vi "reg_visu check 20 client.vi"() -> ()   [LabVIEW 2019]
uses:
  Heating/Global stop.vi
panel:
  out "Array 3":errorcluster[](array[cluster])
  in  "Array 2":string[](array[string])=["GM1", "GM2"]
  out "Errors":errorcluster[](array[cluster])
  out "Progress 3":i32(slide) scale=0.0..20.0
  in  "Stop":bool
  in  "Array":string[](array[string])=["GM1", "GM2", "GM3", "GM4", "GM5", "GM6", "GM7", "GM8", "GM9", "GM10", "GM11", "GM12", "GM13", "GM14", "GM15", "GM16", "GM17", "GM18", "GM19", "GM20"]
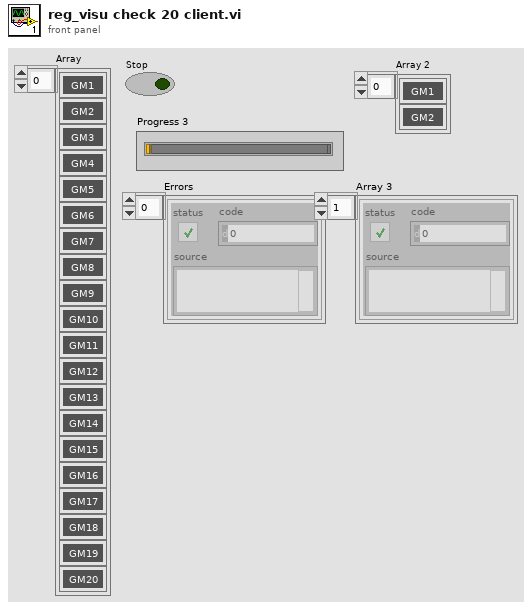
[diagram p1: front panel]
types:
  T1 = enum32{"Invalid", "Standard", "Closed", "Hidden", "Minimized", "Maximized"}
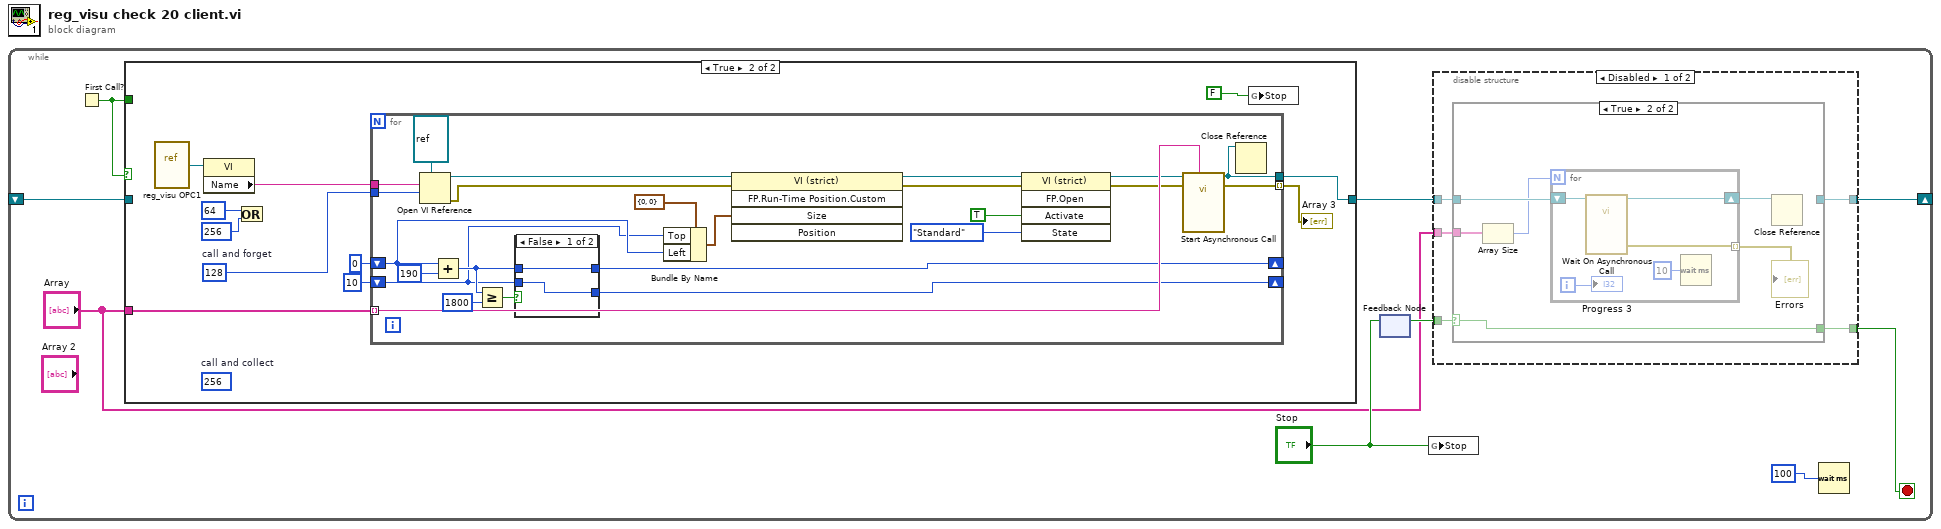
[diagram p0: block diagram]
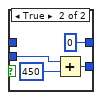
[diagram p5: hidden frame]
diagram:
  n1 = while {
    shift-right: [w5] -> _
    shift-left: _ -> [w7]
    stop <- w2 stop-if-true
    n2 = First Call?() -> (First Call?: T/F=w8:bool)
    n3 = case shown="True" w8 {
      tunnel: w8 -> [_ _]
      tunnel: "Array" -> [_ w39]
      tunnel: [w30 w41] -> w6
      tunnel: w7 -> [w30 _]
      frame False {
      }
      frame True {
        w32 = 128  # call and forget
        (unwired) 256  # call and collect
        n4 = vi-ref "reg_visu OPC1.vi"() -> (w40:refnum<vi>)
        n5 = property class="VI"(reference=w40) -> ("Name"=w33:string)  [unwired: 1 in, 2 out]
        n6 = Or(x=64 ("options"), y=256 ("options")) -> ()  [unwired: 1 out]
        n7 = for {
          tunnel: w39 -> [w65] mode=indexing
          shift-right: [w57] -> _
          shift-left: 0 ("x") -> [w50]
          shift-right: [w56] -> _
          shift-left: 10 ("x") -> [w49]
          tunnel: [w43] -> w41
          tunnel: w32 -> [w47]
          tunnel: w33 -> [w46]
          tunnel: [w42] -> w31 mode=indexing
          n8 = Open VI Reference(type specifier VI Refnum (for type only)=refnum<vi> refnum, vi path=w46, options=w47) -> (vi reference=w44:refnum<vi>, error out=w45:errorcluster)  [unwired: 3 in]
          n9 = Add(x=w50, y=190) -> (x+y=w58:i32)
          n10 = Greater Or Equal?(x=w58, y=1800) -> (x >= y?=w59:bool)
          n11 = case shown="False" w59 {
            tunnel: w58 -> [w66 _]
            tunnel: [w66 0 ("x")] -> w57
            tunnel: w49 -> [w67 w70]
            tunnel: [w67 w69] -> w56
            frame False {
            }
            frame True {
              n12 = Add(x=w70, y=450) -> (x+y=w69:i32)
            }
          }
          n13 = Bundle By Name(cluster=cluster{"Top":i16, "Left":i16} {"Top"=0, "Left"=0} ("Position"), "Top"=w49, "Left"=w50) -> (w55:cluster{"Top":i16, "Left":i16})
          n14 = invoke class="VI (strict)" method="FP.Run-Time Position.Custom"(reference=w44, error in=w45, "Size"=w55) -> (reference out=w54:refnum<vi>, error out=w53:errorcluster)  [unwired: 2 in, 3 out]
          n15 = invoke class="VI (strict)" method="FP.Open"(reference=w54, error in=w53, "Activate"=TRUE ("Activate?"), "State"=T1."Standard") -> (reference out=w52:refnum<vi>, error out=w51:errorcluster)  [unwired: 1 in, 3 out]
          n16 = call-by-ref "Start Asynchronous Call"(reference=w52, error in=w51, "name"=w65) -> (reference out=w43:refnum<vi>, error out=w42:errorcluster)  [unwired: 9 in, 2 out]
          n17 = Close Reference(reference=w43) -> ()  [unwired: 1 in, 1 out]
        }
        "Array 3" <- w31
        n18 = global write "Global stop.vi" "Stop"(FALSE ("Stop")) -> ()
      }
    }
    n19 = feedback-in #1("Stop") -> ()
    n20 = feedback #1() -> (w4:bool)  [unwired: 1 in]
    n21 = global write "Global stop.vi" "Stop"("Stop") -> ()
    n22 = disable-structure shown="Disabled" {
      disable-tunnel: w6 -> [w14 w28]
      disable-tunnel: [w13 w28] -> w5
      disable-tunnel: "Array" -> [w12 _]
      disable-tunnel: w4 -> [w11 w29]
      disable-tunnel: [w10 w29] -> w2
      frame Disabled {
        n23 = case shown="True" w11 {
          selector: w11 -> [w15 w17]
          tunnel: w14 -> [w16 w22]
          tunnel: [w16 _] -> w13
          tunnel: w12 -> [_ w21]
          tunnel: [w15 w17] -> w10
          frame False {
          }
          frame True {
            n24 = Array Size(array=w21) -> (size(s)=w20:i32)
            n25 = for {
              N: w20 -> [_]
              shift-right: [w25] -> w19
              shift-left: w22 -> [w26]
              tunnel: [w24] -> w18 mode=indexing
              i -> [w27]
              n26 = call-by-ref "Wait On Asynchronous Call"(reference=w26) -> (reference out=w25:refnum<vi>, "error out"=w24:errorcluster)  [unwired: 11 in, 2 out]
              n27 = Wait (ms)(milliseconds to wait=u32 10) -> ()  [unwired: 1 out]
              "Progress 3" <- w27
            }
            "Errors" <- w18
            n28 = Close Reference(reference=w19) -> ()  [unwired: 1 in, 1 out]
          }
        }
      }
      frame Enabled {
      }
    }
    n29 = Wait (ms)(milliseconds to wait=u32 100) -> ()  [unwired: 1 out]
  }
